vi "Actor Core.vi"(8 "error in":errorcluster, 11 "Timing Engine in":refnum<class "Timing Engine.lvclass">) -> (0 "error out":errorcluster, 3 "Actor out":refnum<class "Actor.lvclass">)   [LabVIEW 2016, in "Assert API Components.lvlib" / "Assert Display.lvlib" / "Timing Engine.lvlib" / "Timing Engine.lvclass"]
doc: "(<B>Filename</B>: Actor Framework.lvlib:Actor.lvclass:Actor Core.vi)\n\nReceives messages to the actor, reacts to them, and initiates any error handling that may shut the actor down.\n\nDescendant classes may override this VI to append parallel tasks for the actor to complete while it handles messages. Overrides use the Call Parent Method node."
uses:
  Timing Engine.lvclass
  D:/Work/Projects/Actor_Assert_API/Base UI Actor/Base UI Actor/Base UI Actor.lvclass
  C:/Program Files (x86)/National Instruments/LabVIEW 2016/vi.lib/ActorFramework/Actor/Actor.lvclass
  <vilib>/ActorFramework/Actor/Actor.lvclass
  <vilib>/ActorFramework/Actor/Actor.lvclass/Actor.ctl
  Base UI Actor/Base UI Actor/Base UI Actor.lvclass/Base UI Actor.ctl
  Timing Engine.lvclass/Timing Engine.ctl
  <vilib>/ActorFramework/Message Enqueuer/Message Enqueuer.lvclass/Message Enqueuer.ctl
  <vilib>/ActorFramework/Message Enqueuer/Enqueue.vi
  Main Display/Main Display Messages/Update UI Msg/Update UI Msg.lvclass
  C:/Program Files (x86)/National Instruments/LabVIEW 2016/vi.lib/ActorFramework/Message/Message.lvclass
  <vilib>/ActorFramework/Message Priority Queue/Priority Enqueue.vi
  Base UI Actor/Base UI Actor/Base UI Actor.lvclass
panel:
  out "Count":i32
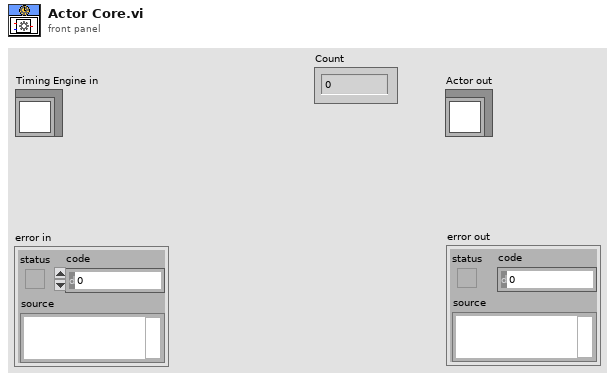
[diagram p1: front panel]
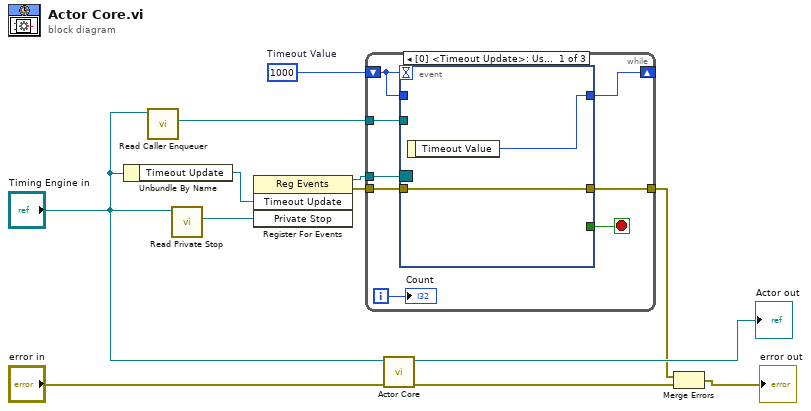
[diagram p0: block diagram]
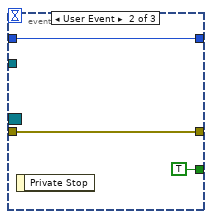
[diagram p2: hidden frame]
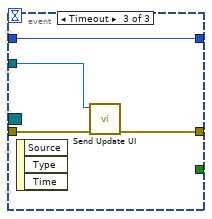
[diagram p3: hidden frame]
diagram:
  w8 = 1000  # Timeout Value
  n1 = Unbundle By Name("Timing Engine in") -> ("Timeout Update"=w10:refnum<user-event>)
  n2 = call <vilib>:"Read Caller Enqueuer.vi"("Actor"="Timing Engine in") -> ("Caller Enqueuer"=w1:refnum<class "Message Enqueuer.lvclass">)  [unwired: 10 in]
  n3 = call "Read Private Stop.vi"("Base UI Actor in"="Timing Engine in") -> ("Private Stop"=w7:refnum<user-event>)  [unwired: 10 in]
  n4 = register-events(w10, w7) -> (reference out=w9:refnum<event-registration>, error out=w6:errorcluster)  [unwired: 2 in]
  n5 = while {
    shift-right: [w19] -> _
    shift-left: w8 -> [w18]
    tunnel: w9 -> [w20]
    tunnel: w6 -> [w16]
    tunnel: [w15] -> w3
    tunnel: w1 -> [w13]
    i -> [w14]
    stop <- w17 stop-if-true
    n6 = event shown="[0] <Timeout Update>: User Event" {
      selector: w20 -> [_ _ _]
      dyn-events: _ -> [_ _ _]
      timeout: w18 -> [_ _ _]
      tunnel: [w22 w23 w29] -> w19
      tunnel: w18 -> [_ w23 w29]
      tunnel: [_ TRUE _] -> w17
      tunnel: w16 -> [w21 w25 w28]
      tunnel: [w21 w25 w27] -> w15
      tunnel: w13 -> [_ _ w26]
      event User Event {
        n7 = event-data() -> ("Timeout Value"=w22:i32)  [unwired: 1 in]
      }
      event User Event {
        n8 = event-data() -> ()  [unwired: 1 in, 1 out]
      }
      event Timeout {
        n9 = event-data() -> ()  [unwired: 1 in, 3 out]
        n10 = call "Send Update UI.vi"("error in (no error)"=w28, "Message Enqueuer"=w26) -> ("error out"=w27:errorcluster)  [unwired: 8 in, 1 out]
      }
    }
    "Count" <- w14
  }
  n11 = call-parent "Actor Core.vi"("error in"="error in", "Actor in"="Timing Engine in") -> ("error out"=w12:errorcluster, "Actor out"=→"Actor out":refnum<class "Actor.lvclass">)  [unwired: 8 in]
  n12 = Merge Errors(w3, w12) -> (→"error out":errorcluster)
